vi "Pack for gRPC.vi"(8 "error in":errorcluster, 9 "configuration / results":enum16{"Configuration", "Results"}(ring), 10 "data value":variant, 11 "measurement customizations in":refnum<class "Measurement Plugin.lvclass">) -> (0 "error out":errorcluster, 2 "any":T1, 3 "measurement customizations out":refnum<class "Measurement Plugin.lvclass">)   [LabVIEW 2020, in "Waveform Measurement.lvlib" / "Measurement Plugin.lvclass"]
uses:
  Measurement Plugin.lvclass
  <vilib>/gRPC/LabVIEW gRPC Library/Shared/Any.ctl
  C:/Program Files/National Instruments/LabVIEW 2020/vi.lib/MeasurementLink/MeasurementLink Measurement Server/Measurement Plugin Service/Measurement Plugin Service.lvclass
  Measurement Configuration.ctl
  Measurement Results.ctl
  <vilib>/gRPC/Generated APIs/ni/protobuf/types/RPC Messages/ni_protobuf_types_DoubleAnalogWaveform_Flat.ctl
  <vilib>/gRPC/Generated APIs/ni/protobuf/types/RPC Messages/ni_protobuf_types_PrecisionTimestamp_Flat.ctl
  <vilib>/gRPC/Generated APIs/ni/protobuf/types/RPC Messages/ni_protobuf_types_DoubleAnalogWaveform_AttributesEntry_Flat.ctl
  <vilib>/gRPC/Generated APIs/ni/protobuf/types/RPC Messages/ni_protobuf_types_WaveformAttributeValue_Flat.ctl
  2eca732d-dbaa-43bf-a7dd-ede2da65bc1b.vi
  a6012965-5700-4384-8228-972e71b6560c.vi
  <vilib>/gRPC/LabVIEW gRPC Library/Server API/Translate Protobuf Error.vi
  <vilib>/AdvancedString/1D String Array to Delimited String.vi
  <vilib>/gRPC/LabVIEW gRPC Library/Server API/Server/Get Server DLL Path.vi
  Waveform Measurement.lvlib
  <vilib>/MeasurementLink/MeasurementLink Measurement Server/Measurement Plugin Service/Measurement Plugin Service.lvclass
  <vilib>/gRPC/Generated APIs/ni/protobuf/types/ni.protobuf.types.lvlib
  <vilib>/gRPC/LabVIEW gRPC Library/grpc-lvsupport-release.lvlib
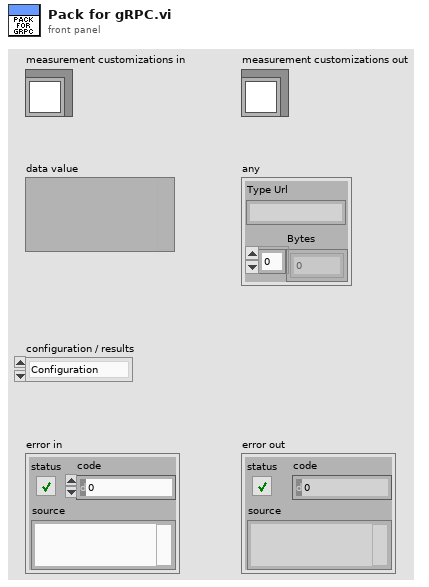
[diagram p1: front panel]
types:
  T1 = typedef "grpc-lvsupport-release.lvlib/Any.ctl" = cluster{"Type Url":string, "Bytes":u8[]}
  T2 = typedef "grpc-lvsupport-release.lvlib/grpcId.ctl" = u64
  T3 = typedef "Waveform Measurement.lvlib/Measurement Configuration.ctl" = cluster{"Signal Type":enum32{"Sinewave", "Triangle", "Square", "Sawtooth"}, "Number of Samples":u32, "Amplitude":dbl, "Frequency":dbl, "Sample Rate":u32, "Offset":dbl}
  T4 = typedef "Waveform Measurement.lvlib/Measurement Results.ctl" = cluster{"Waveform":T5}
  T5 = typedef "ni.protobuf.types.lvlib/ni_protobuf_types_DoubleAnalogWaveform_Flat.ctl" = cluster{"t0":T6, "dt":dbl, "y_data":dbl[], "attributes":T7[]}
  T6 = typedef "ni.protobuf.types.lvlib/ni_protobuf_types_PrecisionTimestamp_Flat.ctl" = cluster{"seconds":i64, "fractional_seconds":u64}
  T7 = typedef "ni.protobuf.types.lvlib/ni_protobuf_types_DoubleAnalogWaveform_AttributesEntry_Flat.ctl" = cluster{"key":string, "value":T8}
  T8 = typedef "ni.protobuf.types.lvlib/ni_protobuf_types_WaveformAttributeValue_Flat.ctl" = cluster{"ni_protobuf_types_WaveformAttributeValue_attribute_selected_index":i32, "bool_value":bool, "integer_value":i32, "double_value":dbl, "string_value":string}
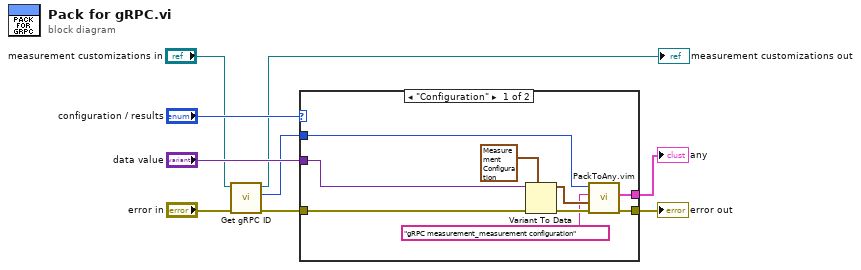
[diagram p0: block diagram]
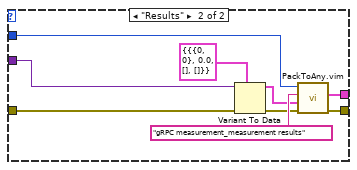
[diagram p2: hidden frame]
diagram:
  n1 = call <vilib>:"Get gRPC ID.vi"("error in"="error in", "measurement plugin service in"="measurement customizations in") -> ("error out"=w4:errorcluster, "gRPC ID"=w1:T2, "measurement plugin service out"=→"measurement customizations out":refnum<class "Measurement Plugin.lvclass">)  [unwired: 7 in]
  n2 = case shown="\"Configuration\"" "configuration / results" {
    tunnel: w4 -> [w18 w27]
    tunnel: "data value" -> [w17 w26]
    tunnel: w1 -> [w14 w22]
    tunnel: [w16 w24] -> w8
    tunnel: [w15 w23] -> w7
    frame "Configuration" {
      n3 = Variant To Data(error in=w18, type=T3 {"Signal Type"=enum."Sawtooth", "Number of Samples"=32, "Amplitude"=32.0, "Frequency"=64.0, "Sample Rate"=64, "Offset"=-32.0} ("measurement configuration"), Variant=w17) -> (data=w13:T3, error out=w12:errorcluster)
      n4 = call "PackToAny.vim"("error in"=w12, "Data To Pack"=w13, "Message Type"="gRPC measurement_measurement configuration", "gRPCid in"=w14) -> ("error out"=w16:errorcluster, "Any"=w15:T1)  [unwired: 5 in, 1 out]
    }
    frame "Results" {
      n5 = Variant To Data(error in=w27, type=T4 {"Waveform"={"t0"={"seconds"=0, "fractional_seconds"=0}, "dt"=0.0, "y_data"=[], "attributes"=[]}} ("Measurement Results"), Variant=w26) -> (data=w20:T4, error out=w19:errorcluster)
      n6 = call "PackToAny.vim"("error in"=w19, "Data To Pack"=w20, "Message Type"="gRPC measurement_measurement results", "gRPCid in"=w22) -> ("error out"=w24:errorcluster, "Any"=w23:T1)  [unwired: 5 in, 1 out]
    }
  }
  "error out" <- w8
  "any" <- w7
